vi "tethered test.vi"   [LabVIEW 2012, in "Omni2013.lvrbt"]
uses:
  Omni2013.lvrbt
  <vilib>/NXT/Dual Mode Library/Display/drawNumber_float.vi
types:
  T1 = typedef "FTC ControllerState.ctl" = cluster{"Left X":i8, "Left Y":i8, "Right X":i8, "Right Y":i8, "Button Encoding 9-12":u8, "Button Encoding 1-8":u8, "POV":T2}
  T2 = typedef "FTC POVState.ctl" = i8
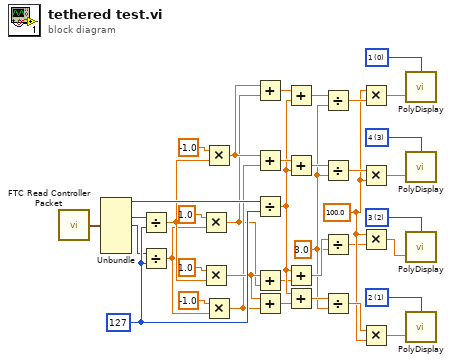
[diagram p0: block diagram]
diagram:
  w1 = i16 0 items=["1", "2", "3", "4", "5", "6", "7", "8"] ("Line")
  w3 = i16 3 items=["1", "2", "3", "4", "5", "6", "7", "8"] ("Line")
  w6 = i16 2 items=["1", "2", "3", "4", "5", "6", "7", "8"] ("Line")
  w7 = i16 1 items=["1", "2", "3", "4", "5", "6", "7", "8"] ("Line")
  w14 = 100.0 ("y")
  w9 = 3.0 ("y")
  w37 = i8 127 ("y")
  n1 = call <vilib>:"FTC Read Controller Packet.vi"() -> ("Controller State"=w12:T1)  [unwired: 5 in]
  n2 = Unbundle(w12) -> ("Left X"=w38:i8, "Right X"=w35:i8, "Right Y"=w36:i8)  [unwired: 4 out]
  n3 = Divide(x=w35, y=w37) -> (x/y=w32:dbl)
  n4 = Divide(x=w36, y=w37) -> (x/y=w29:dbl)
  n5 = Multiply(x=1.0, y=w29) -> (x*y=w11:dbl)
  n6 = Multiply(x=1.0, y=w32) -> (x*y=w28:dbl)
  n7 = Multiply(x=-1.0, y=w32) -> (x*y=w27:dbl)
  n8 = Multiply(x=-1.0, y=w29) -> (x*y=w26:dbl)
  n9 = Add(x=w27, y=w11) -> (x+y=w23:dbl)
  n10 = Add(x=w27, y=w26) -> (x+y=w25:dbl)
  n11 = Divide(x=w38, y=w37) -> (x/y=w19:dbl)
  n12 = Add(x=w28, y=w11) -> (x+y=w10:dbl)
  n13 = Add(x=w28, y=w26) -> (x+y=w24:dbl)
  n14 = Add(x=w23, y=w19) -> (x+y=w22:dbl)
  n15 = Add(x=w25, y=w19) -> (x+y=w20:dbl)
  n16 = Add(x=w19, y=w10) -> (x+y=w18:dbl)
  n17 = Add(x=w19, y=w24) -> (x+y=w21:dbl)
  n18 = Divide(x=w22, y=w9) -> (x/y=w15:dbl)
  n19 = Divide(x=w20, y=w9) -> (x/y=w17:dbl)
  n20 = Divide(x=w18, y=w9) -> (x/y=w8:dbl)
  n21 = Divide(x=w21, y=w9) -> (x/y=w16:dbl)
  n22 = Multiply(x=w14, y=w15) -> (x*y=w2:dbl)
  n23 = Multiply(x=w17, y=w14) -> (x*y=w4:dbl)
  n24 = Multiply(x=w14, y=w8) -> (x*y=w5:dbl)
  n25 = Multiply(x=w16, y=w14) -> (x*y=w13:dbl)
  n26 = call-poly <vilib>:"PolyDisplay.vi"("number"=w2, "Line"=w1) -> ()  [unwired: 2 in, 1 out]
  n27 = call-poly <vilib>:"PolyDisplay.vi"("number"=w4, "Line"=w3) -> ()  [unwired: 2 in, 1 out]
  n28 = call-poly <vilib>:"PolyDisplay.vi"("number"=w5, "Line"=w6) -> ()  [unwired: 2 in, 1 out]
  n29 = call-poly <vilib>:"PolyDisplay.vi"("number"=w13, "Line"=w7) -> ()  [unwired: 2 in, 1 out]
